vi "Update.vi"(2 "error in (no error)":errorcluster, 3 "Time Since Last Update":dbl, 4 "Car.lvclass":refnum<class "Car.lvclass">) -> (0 "error out":errorcluster, 1 "Car.lvclass 2":refnum<class "Car.lvclass">)   [LabVIEW 2015, in "Car.lvclass"]
uses:
  Car.lvclass
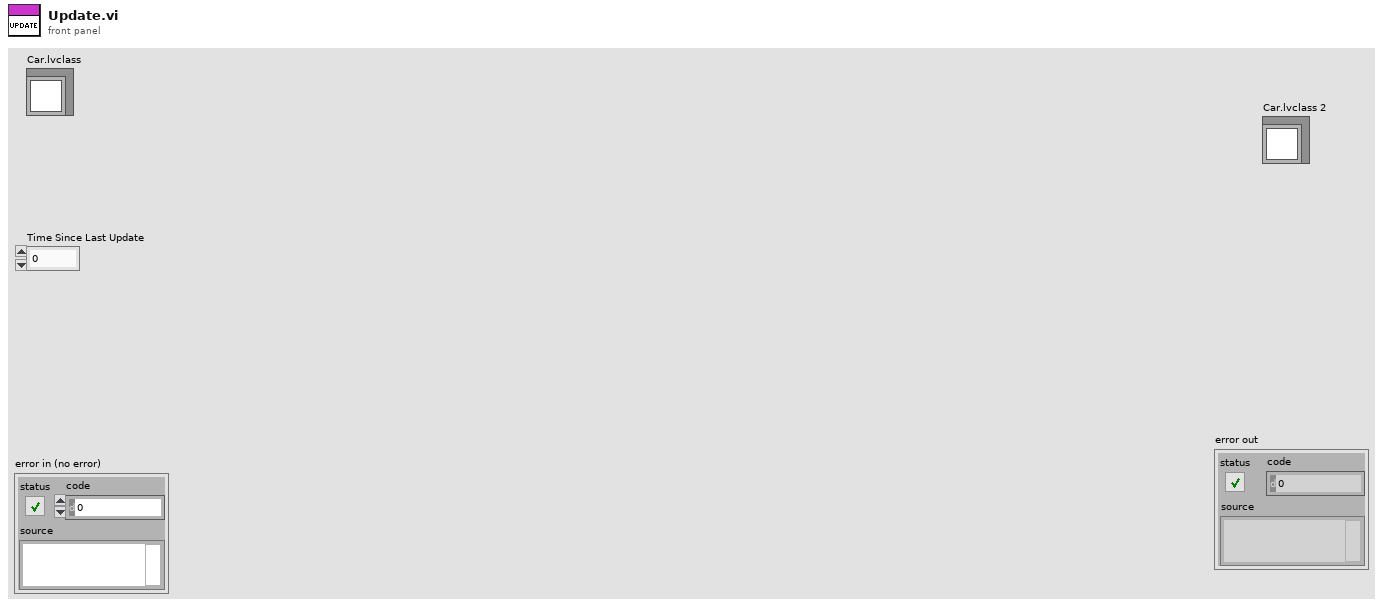
[diagram p1: front panel]
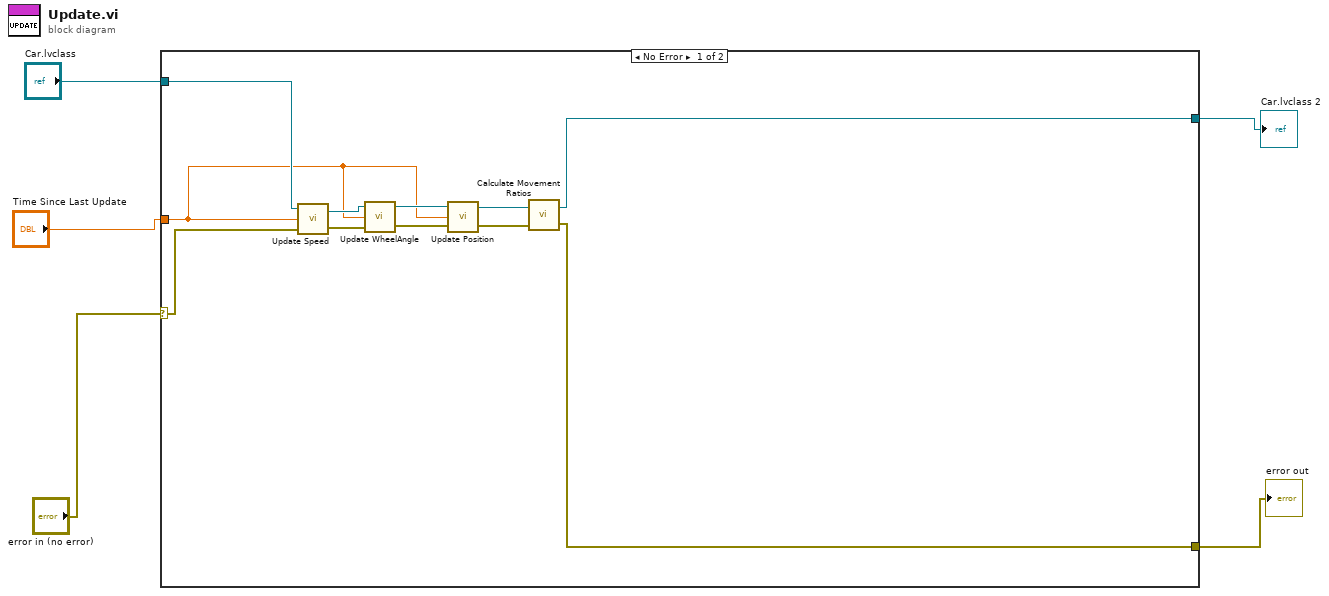
[diagram p0: block diagram]
diagram:
  n1 = case shown="No Error" "error in (no error)" {
    selector: "error in (no error)" -> [w15 w18]
    tunnel: [w6 w18] -> w4
    tunnel: [w7 w17] -> w3
    tunnel: "Car.lvclass" -> [w16 w17]
    tunnel: "Time Since Last Update" -> [w10 _]
    frame No Error {
      n2 = call "Update Speed.vi"("error in (no error)"=w15, "Time Since Last Update"=w10, "Car.lvclass"=w16) -> ("error out"=w13:errorcluster, "Car.lvclass 2"=w14:refnum<class "Car.lvclass">)
      n3 = call "Update WheelAngle.vi"("error in (no error)"=w13, "Time Since Last Update"=w10, "Car.lvclass"=w14) -> ("error out"=w11:errorcluster, "Car.lvclass 2"=w12:refnum<class "Car.lvclass">)
      n4 = call "Update Position.vi"("error in (no error)"=w11, "Time Since Last Update"=w10, "Car.lvclass"=w12) -> ("error out"=w8:errorcluster, "Car.lvclass 2"=w9:refnum<class "Car.lvclass">)
      n5 = call "Calculate Movement Ratios.vi"("error in (no error)"=w8, "Car.lvclass"=w9) -> ("error out"=w6:errorcluster, "Car.lvclass 2"=w7:refnum<class "Car.lvclass">)
    }
    frame Error {
    }
  }
  "Car.lvclass 2" <- w3
  "error out" <- w4
